vi "begin_ShootDualTallonSrxl.vi"(4 "Time":T1, 5 "Enc Edges / Rev":dbl=1440.0 format="%.4f", 6 "Distance Type":T2, 7 "MAX DESIRED\nVELOCITY\n(UNITS)":dbl=5800.0 format="%#_13g", 8 "Wheel Radius In":dbl=3.0 format="%.4f", 9 "Left Master CAN":u8=14, 11 "RIght Master CAN":u8=10) -> ()   [LabVIEW 2019, in "ShootDualTalonSRX_Motor_Pair.lvlib"]
doc: "Open drives for 4 motor arcade drive using Talon SRX controllers. Configure for velocity control using directly wired encoders on master talon."
uses:
  ShootDualTalonSRX_Motor_Pair.lvlib
  Dist_Type.ctl
  Time_Units_Control.ctl
  <vilib>/Rock Robotics/WPI/ThirdParty/Phoenix-LabVIEW/Motor Controller/Controls/CTRE_Phoenix_MotorControl_FeedbackDevice.ctl
  <vilib>/Rock Robotics/WPI/ThirdParty/Phoenix-LabVIEW/Motor Controller/Controls/CTRE_Phoenix_MotorControl_NeutralMode.ctl
  globals_ShootDualTalonSRX.vi
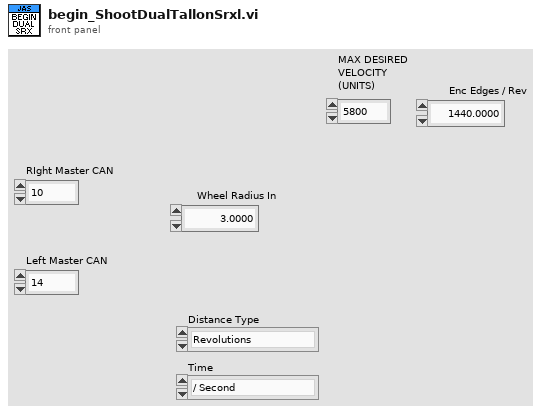
[diagram p1: front panel]
types:
  T1 = typedef "ShootDualTalonSRX_Motor_Pair.lvlib/Time_Units_Control.ctl" = enum16{"/ Second", "/ Minute"}
  T2 = typedef "ShootDualTalonSRX_Motor_Pair.lvlib/Dist_Type.ctl" = enum16{"Revolutions", "Feet"}
  T3 = typedef "CTRE_Phoenix_MotorControl_FeedbackDevice.ctl" = i8
  T4 = typedef "CTRE_Phoenix_MotorControl_NeutralMode.ctl" = enum8{"EEPROMSetting", "Override to Coast", "Override to Brake"}
  T5 = typedef "WPI_MotorControlDeviceRef.ctl" = cluster{"DeviceStatus":errorcluster, "Type":T6, "PWM":cluster{"PWM Channel":T7, "DeadBand":T8}, "CAN":cluster{"Device Number":u8, "SetOutput VI Ref":variant, "GetOutput VI Ref":variant, "Enable VI Ref":variant, "Disable VI Ref":variant, "Data":variant}, "Invert":bool, "DIO PWM":cluster{"PWM \"Enable\" Channel":T7, "DIOChannel":T9, "PWM Rate":dbl}}
  T6 = typedef "WPI_MotorControlType.ctl" = enum16{"PWM", "CAN", "DIO PWM"}
  T7 = typedef "FPGA_DIOPWMChannel.ctl" = enum8{"PWM 0", "PWM 1", "PWM 2", "PWM 3", "PWM 4", "PWM 5", "PWM 6", "PWM 7", "PWM 8", "PWM 9", "PWM MXP 0", "PWM MXP 1", "PWM MXP 2", "PWM MXP 3", "PWM MXP 4", "PWM MXP 5", "PWM MXP 6", "PWM MXP 7", "PWM MXP 8", "PWM MXP 9", "Invalid"}
  T8 = typedef "WPI_PWMDeadband.ctl" = cluster{"Name":string, "maxPositivePwm":i32, "minPositivePwm":i32, "centerPwm":i32, "maxNegativePwm":i32, "minNegativePwm":i32, "angularRange":u16}
  T9 = typedef "FPGA_DIOChannel.ctl" = enum8{"DIO 0", "DIO 1", "DIO 2", "DIO 3", "DIO 4", "DIO 5", "DIO 6", "DIO 7", "DIO 8", "DIO 9", "DIO MXP 0", "DIO MXP 1", "DIO MXP 2", "DIO MXP 3", "DIO MXP 4", "DIO MXP 5", "DIO MXP 6", "DIO MXP 7", "DIO MXP 8", "DIO MXP 9", "DIO MXP 10", "DIO MXP 11", "DIO MXP 12", "DIO MXP 13", "DIO MXP 14", "DIO MXP 15", "SPI Port CS1", "SPI Port CS2", "SPI Port CS3", "SPI Port MISO", "SPI Port MOSI", "Invalid"}
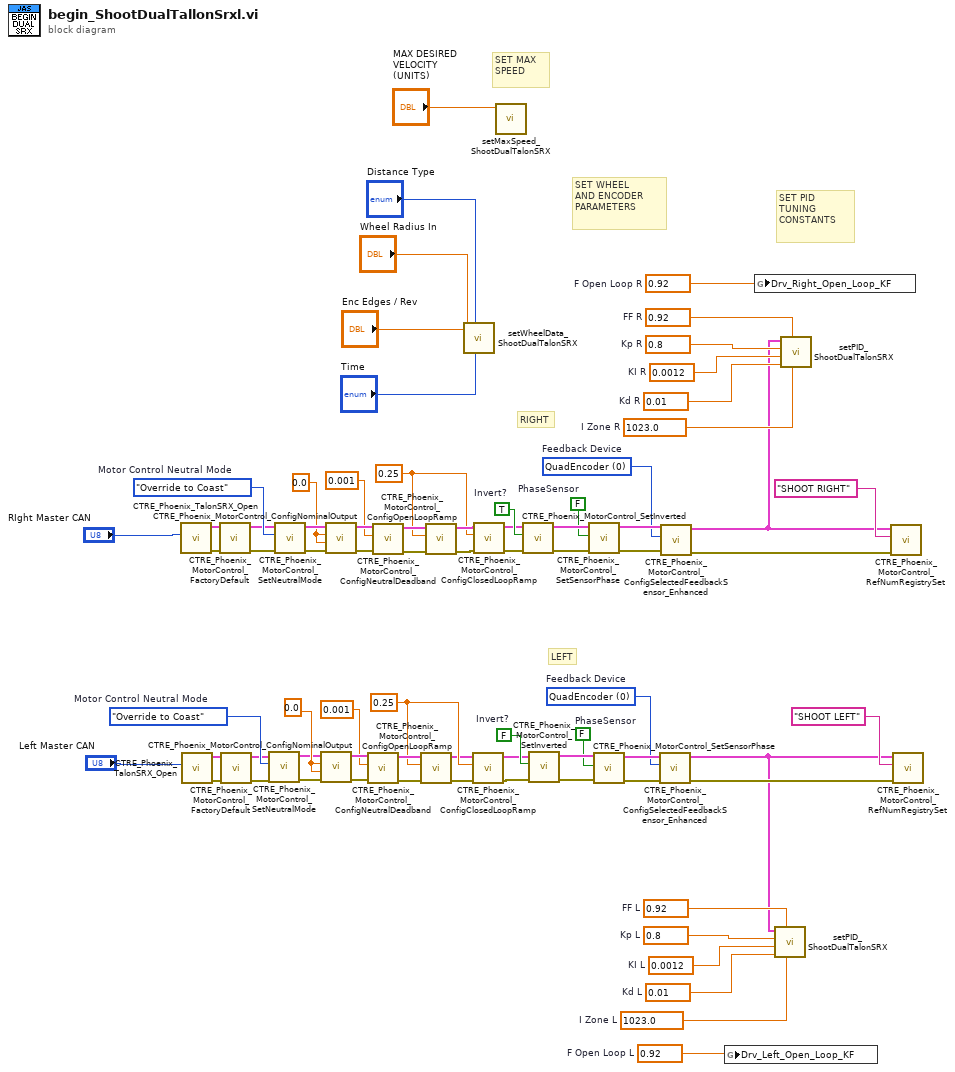
[diagram p0: block diagram]
diagram:
  w5 = 0.25 ("secondsFromNeutralToFull")
  w11 = 0.0 ("Forward Nominal Percent Output")
  w14 = 0.25 ("secondsFromNeutralToFull")
  w22 = 0.0 ("Forward Nominal Percent Output")
  w33 = 0.92  # F Open Loop L
  w41 = 1023.0  # I Zone L
  w42 = 0.01  # Kd L
  w43 = 0.0012  # KI L
  w44 = 0.8  # Kp L
  w45 = 0.92  # FF L
  w35 = 1023.0  # I Zone R
  w36 = 0.01  # Kd R
  w37 = 0.0012  # KI R
  w38 = 0.8  # Kp R
  w39 = 0.92  # FF R
  w32 = 0.92  # F Open Loop R
  w46 = FALSE  # Invert?
  w71 = TRUE  # Invert?
  w64 = T3 0 items=["None"=-1, "QuadEncoder"=0, "Analog"=2, "Tachometer"=4, "Pulse Width Encoded Position"=8, "Sensor Sum (S0 + S1)"=9, "Sensor Difference (D0 - D1)"=10, "Remote Source 0"=11, "Remote Source 1"=12, "Software Emulated"=15]  # Feedback Device
  w63 = T3 0 items=["None"=-1, "QuadEncoder"=0, "Analog"=2, "Tachometer"=4, "Pulse Width Encoded Position"=8, "Sensor Sum (S0 + S1)"=9, "Sensor Difference (D0 - D1)"=10, "Remote Source 0"=11, "Remote Source 1"=12, "Software Emulated"=15]  # Feedback Device
  w62 = CTRE_Phoenix_MotorControl_NeutralMode."Override to Coast"  # Motor Control Neutral Mode
  w59 = CTRE_Phoenix_MotorControl_NeutralMode."Override to Coast"  # Motor Control Neutral Mode
  w54 = FALSE  # PhaseSensor
  w49 = FALSE  # PhaseSensor
  # "SET PID\nTUNING\nCONSTANTS"
  # "SET WHEEL\nAND ENCODER\nPARAMETERS"
  # "SET MAX\nSPEED"
  # "RIGHT"
  # "LEFT"
  n1 = call <vilib>:"CTRE_Phoenix_TalonSRX_Open.vi"("Device Number"="RIght Master CAN") -> ("error out"=w56:errorcluster, "CAN Talon SRX Ref"=w55:T5)  [unwired: 9 in]
  n2 = call <vilib>:"CTRE_Phoenix_TalonSRX_Open.vi"("Device Number"="Left Master CAN") -> ("error out"=w51:errorcluster, "CAN Talon SRX Ref"=w50:T5)  [unwired: 9 in]
  n3 = call <vilib>:"CTRE_Phoenix_MotorControl_FactoryDefault.vi"("error in"=w56, "PhoenixMotorControlDevRef"=w55) -> ("error out"=w61:errorcluster, "PhoenixMotorControlDevRef"=w60:T5)  [unwired: 8 in]
  n4 = call <vilib>:"CTRE_Phoenix_MotorControl_FactoryDefault.vi"("error in"=w51, "PhoenixMotorControlDevRef"=w50) -> ("error out"=w58:errorcluster, "PhoenixMotorControlDevRef"=w57:T5)  [unwired: 8 in]
  n5 = call <vilib>:"CTRE_Phoenix_MotorControl_SetNeutralMode.vi"("error in (no error)"=w58, "Motor Control Neutral Mode"=w59, "PhoenixMotorControlDevRef"=w57) -> ("error out"=w6:errorcluster, "PhoenixMotorControlDevRef"=w7:T5)  [unwired: 7 in]
  n6 = call <vilib>:"CTRE_Phoenix_MotorControl_SetNeutralMode.vi"("error in (no error)"=w61, "Motor Control Neutral Mode"=w62, "PhoenixMotorControlDevRef"=w60) -> ("error out"=w26:errorcluster, "PhoenixMotorControlDevRef"=w25:T5)  [unwired: 7 in]
  n7 = call <vilib>:"CTRE_Phoenix_MotorControl_ConfigNominalOutput.vi"("error in (no error)"=w6, "Reverse Nominal Percent Output"=w11, "Forward Nominal Percent Output"=w11, "PhoenixMotorControlDevRef"=w7) -> ("error out"=w9:errorcluster, "PhoenixMotorControlDevRef"=w10:T5)  [unwired: 6 in]
  n8 = call <vilib>:"CTRE_Phoenix_MotorControl_ConfigNominalOutput.vi"("error in (no error)"=w26, "Reverse Nominal Percent Output"=w22, "Forward Nominal Percent Output"=w22, "PhoenixMotorControlDevRef"=w25) -> ("error out"=w20:errorcluster, "PhoenixMotorControlDevRef"=w21:T5)  [unwired: 6 in]
  n9 = call <vilib>:"CTRE_Phoenix_MotorControl_ConfigNeutralDeadband.vi"("error in (no error)"=w9, "Percent Deadband"=0.001, "PhoenixMotorControlDevRef"=w10) -> ("error out"=w13:errorcluster, "PhoenixMotorControlDevRef"=w12:T5)  [unwired: 7 in]
  n10 = call <vilib>:"CTRE_Phoenix_MotorControl_ConfigNeutralDeadband.vi"("error in (no error)"=w20, "Percent Deadband"=0.001, "PhoenixMotorControlDevRef"=w21) -> ("error out"=w24:errorcluster, "PhoenixMotorControlDevRef"=w23:T5)  [unwired: 7 in]
  n11 = call <vilib>:"CTRE_Phoenix_MotorControl_ConfigOpenLoopRamp.vi"("error in (no error)"=w13, "secondsFromNeutralToFull"=w5, "PhoenixMotorControlDevRef"=w12) -> ("error out"=w1:errorcluster, "PhoenixMotorControlDevRef"=w4:T5)  [unwired: 7 in]
  n12 = call <vilib>:"CTRE_Phoenix_MotorControl_ConfigOpenLoopRamp.vi"("error in (no error)"=w24, "secondsFromNeutralToFull"=w14, "PhoenixMotorControlDevRef"=w23) -> ("error out"=w15:errorcluster, "PhoenixMotorControlDevRef"=w16:T5)  [unwired: 7 in]
  n13 = call "setWheelData_ShootDualTalonSRX.vi"("Time"="Time", "Distance Type"="Distance Type", "Enc Edges / Rev"="Enc Edges / Rev", "Wheel Radius In"="Wheel Radius In") -> ()  [unwired: 3 in, 5 out]
  n14 = call <vilib>:"CTRE_Phoenix_MotorControl_ConfigClosedLoopRamp.vi"("error in (no error)"=w1, "secondsFromNeutralToFull"=w5, "PhoenixMotorControlDevRef"=w4) -> ("error out"=w2:errorcluster, "PhoenixMotorControlDevRef"=w3:T5)  [unwired: 7 in]
  n15 = call <vilib>:"CTRE_Phoenix_MotorControl_ConfigClosedLoopRamp.vi"("error in (no error)"=w15, "secondsFromNeutralToFull"=w14, "PhoenixMotorControlDevRef"=w16) -> ("error out"=w18:errorcluster, "PhoenixMotorControlDevRef"=w17:T5)  [unwired: 7 in]
  n16 = call "setMaxSpeed_ShootDualTalonSRX.vi"("MAX DESIRED\nVELOCITY (UNITS)"="MAX DESIRED\nVELOCITY\n(UNITS)") -> ()  [unwired: 8 in, 2 out]
  n17 = call <vilib>:"CTRE_Phoenix_MotorControl_SetInverted.vi"("error in (no error)"=w18, "Invert?"=w71, "PhoenixMotorControlDevRef"=w17) -> ("error out"=w70:errorcluster, "PhoenixMotorControlDevRef"=w69:T5)  [unwired: 7 in]
  n18 = call <vilib>:"CTRE_Phoenix_MotorControl_SetInverted.vi"("error in (no error)"=w2, "Invert?"=w46, "PhoenixMotorControlDevRef"=w3) -> ("error out"=w66:errorcluster, "PhoenixMotorControlDevRef"=w65:T5)  [unwired: 7 in]
  n19 = call <vilib>:"CTRE_Phoenix_MotorControl_SetSensorPhase.vi"("error in (no error)"=w70, "PhaseSensor"=w54, "PhoenixMotorControlDevRef"=w69) -> ("error out"=w72:errorcluster, "PhoenixMotorControlDevRef"=w73:T5)  [unwired: 7 in]
  n20 = call <vilib>:"CTRE_Phoenix_MotorControl_SetSensorPhase.vi"("error in (no error)"=w66, "PhaseSensor"=w49, "PhoenixMotorControlDevRef"=w65) -> ("error out"=w68:errorcluster, "PhoenixMotorControlDevRef"=w67:T5)  [unwired: 7 in]
  n21 = call <vilib>:"CTRE_Phoenix_MotorControl_ConfigSelectedFeedbackSensor_Enhanced.vi"("error in (no error)"=w68, "Feedback Device"=w64, "PhoenixMotorControlDevRef"=w67) -> ("error out"=w75:errorcluster, "PhoenixMotorControlDevRef"=w40:T5)  [unwired: 7 in]
  n22 = call <vilib>:"CTRE_Phoenix_MotorControl_ConfigSelectedFeedbackSensor_Enhanced.vi"("error in (no error)"=w72, "Feedback Device"=w63, "PhoenixMotorControlDevRef"=w73) -> ("error out"=w74:errorcluster, "PhoenixMotorControlDevRef"=w34:T5)  [unwired: 7 in]
  n23 = global write "globals_ShootDualTalonSRX.vi" "Drv_Left_Open_Loop_KF"(w33) -> ()
  n24 = global write "globals_ShootDualTalonSRX.vi" "Drv_Right_Open_Loop_KF"(w32) -> ()
  n25 = call "setPID_ShootDualTalonSRX.vi"("I ZONE"=w41, "FF"=w45, "KD"=w42, "KI"=w43, "KP"=w44, "MasterDriveRef"=w40) -> ()  [unwired: 6 in]
  n26 = call "setPID_ShootDualTalonSRX.vi"("I ZONE"=w35, "FF"=w39, "KD"=w36, "KI"=w37, "KP"=w38, "MasterDriveRef"=w34) -> ()  [unwired: 6 in]
  n27 = call <vilib>:"CTRE_Phoenix_MotorControl_RefNumRegistrySet.vi"("error in (no error)"=w74, "refnum name"="SHOOT RIGHT", "PhoenixMotorControlDevRef"=w34) -> ()  [unwired: 7 in, 2 out]
  n28 = call <vilib>:"CTRE_Phoenix_MotorControl_RefNumRegistrySet.vi"("error in (no error)"=w75, "refnum name"="SHOOT LEFT", "PhoenixMotorControlDevRef"=w40) -> ()  [unwired: 7 in, 2 out]
